vi "EventDrivenStateMachine.vi"() -> ()   [LabVIEW 2020]
panel:
  in  "Data2Tx":i32
  in  "Stop":bool
  in  "Tx":bool
  out "DataRx":i32
  in  "TxData":T1
  out "error out":errorcluster
  in  "error in":errorcluster
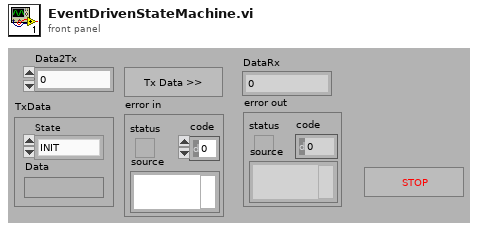
[diagram p1: front panel]
types:
  T1 = cluster{"Data":variant, "State":enum16{"INIT", "TX", "RX", "STOP"}}
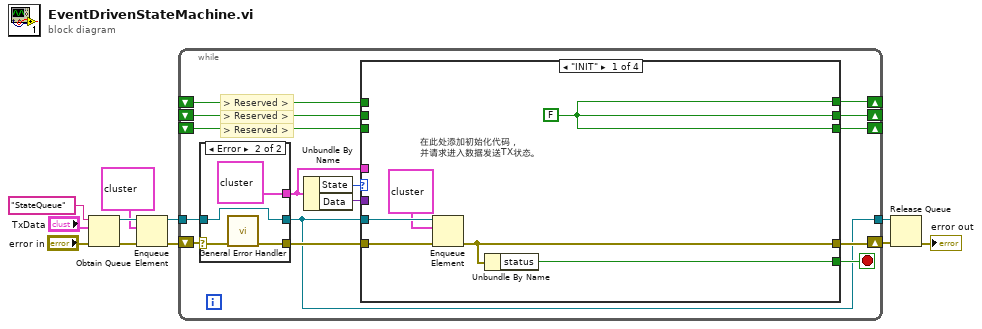
[diagram p0: block diagram]
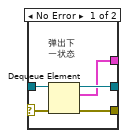
[diagram p2: hidden frame]
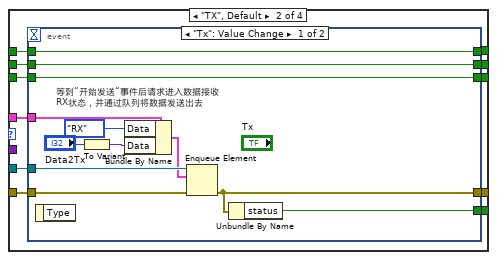
[diagram p3: hidden frame]
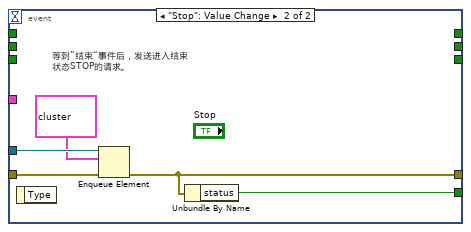
[diagram p4: hidden frame]
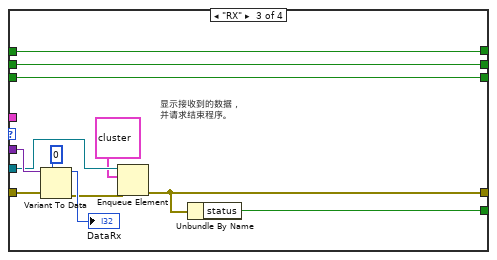
[diagram p5: hidden frame]
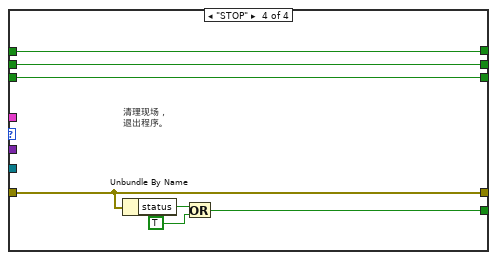
[diagram p6: hidden frame]
diagram:
  n1 = Obtain Queue(name (unnamed)="StateQueue", element data type="TxData", error in (no error)="error in") -> (queue out=w10:refnum<queue>, error out=w9:errorcluster)  [unwired: 2 in, 1 out]
  n2 = Enqueue Element(queue=w10, element=T1 {"Data"=variant, "State"=enum."INIT"} ("Queue Data"), error in (no error)=w9) -> (queue out=w3:refnum<queue>, error out=w2:errorcluster)  [unwired: 1 in, 1 out]
  n3 = while {
    shift-right: [w25] -> w8
    shift-left: w2 -> [w17]
    shift-right: [w21] -> _
    shift-left: _ -> [w19]
    shift-right: [w24] -> _
    shift-left: _ -> [w22]
    shift-right: [w23] -> _
    shift-left: _ -> [w20]
    tunnel: w3 -> [w18]
    tunnel: [w15] -> w7
    stop <- w26 stop-if-true
    # "> Reserved >"
    # "> Reserved >"
    # "> Reserved >"
    n4 = case shown="Error" w17 {
      selector: w17 -> [w30 w35]
      tunnel: w18 -> [w31 w34]
      tunnel: [w29 w34] -> w15
      tunnel: [w28 w33] -> w16
      tunnel: [w27 T1 {"Data"=variant, "State"=enum."RX"} ("Queue Data")] -> w12
      frame No Error {
        # "弹出下\n一状态"
        n5 = Dequeue Element(queue=w31, error in (no error)=w30) -> (queue out=w29:refnum<queue>, element=w27:T1, error out=w28:errorcluster)  [unwired: 1 in, 1 out]
      }
      frame Error {
        n6 = call <vilib>:"General Error Handler.vi"("error in (no error)"=w35) -> ("error out"=w33:errorcluster)  [unwired: 10 in, 4 out]
      }
    }
    n7 = Unbundle By Name(w12) -> ("State"=w14:enum16{"INIT", "TX", "RX", "STOP"}, "Data"=w13:variant)
    n8 = case shown="\"INIT\"" w14 {
      tunnel: [w40 w49 w78 w84] -> w26
      tunnel: w16 -> [w39 w52 w76 w85]
      tunnel: [w38 w50 w70 w85] -> w25
      tunnel: [w41 w43 w80 w87] -> w24
      tunnel: [w41 w42 w81 w86] -> w23
      tunnel: w22 -> [_ w46 w80 w87]
      tunnel: [w41 w44 w79 w88] -> w21
      tunnel: w20 -> [_ w45 w81 w86]
      tunnel: w19 -> [_ w47 w79 w88]
      tunnel: w15 -> [w37 w51 w72 _]
      tunnel: w13 -> [_ _ w77 _]
      tunnel: w12 -> [_ w48 _ _]
      frame "INIT" {
        w41 = FALSE
        # "在此处添加初始化代码，\n并请求进入数据发送TX状态。"
        n9 = Enqueue Element(queue=w37, element=T1 {"Data"=variant, "State"=enum."TX"} ("Queue Data"), error in (no error)=w39) -> (error out=w38:errorcluster)  [unwired: 1 in, 2 out]
        n10 = Unbundle By Name(w38) -> ("status"=w40:bool)
      }
      frame "TX", Default {
        n11 = event shown="[0] \"Tx\": Value Change" {
          selector: _ -> [_ _]
          dyn-events: _ -> [_ _]
          timeout: _ -> [_ _]
          tunnel: w52 -> [w64 w68]
          tunnel: w51 -> [w63 w69]
          tunnel: [w62 w65] -> w50
          tunnel: [w61 w66] -> w49
          tunnel: w48 -> [w60 _]
          tunnel: w47 -> [w57 _]
          tunnel: w46 -> [w56 _]
          tunnel: w45 -> [w55 _]
          tunnel: [w57 _] -> w44
          tunnel: [w56 _] -> w43
          tunnel: [w55 _] -> w42
          event "Tx": Value Change {
            # "等到“开始发送“事件后请求进入数据接收\nRX状态，并通过队列将数据发送出去"
            n12 = event-data() -> ()  [unwired: 1 in, 1 out]
            n13 = To Variant(anything="Data2Tx") -> (Variant=w58:variant)
            n14 = Bundle By Name(cluster=w60, "Data"=enum16{"INIT", "TX", "RX", "STOP"}."RX" ("State"), "Data"=w58) -> (w59:T1)
            n15 = Enqueue Element(queue=w63, element=w59, error in (no error)=w64) -> (error out=w62:errorcluster)  [unwired: 1 in, 2 out]
            n16 = Unbundle By Name(w62) -> ("status"=w61:bool)
          }
          event "Stop": Value Change {
            # "等到”结束“事件后，发送进入结束\n状态STOP的请求。"
            n17 = event-data() -> ()  [unwired: 1 in, 1 out]
            n18 = Enqueue Element(queue=w69, element=T1 {"Data"=variant, "State"=enum."STOP"} ("Queue Data"), error in (no error)=w68) -> (error out=w65:errorcluster)  [unwired: 1 in, 2 out]
            n19 = Unbundle By Name(w65) -> ("status"=w66:bool)
          }
        }
      }
      frame "RX" {
        # "显示接收到的数据，\n并请求结束程序。"
        n20 = Variant To Data(error in=w76, type=0, Variant=w77) -> (data=→"DataRx":i32, error out=w73:errorcluster)
        n21 = Enqueue Element(queue=w72, element=T1 {"Data"=variant, "State"=enum."TX"} ("Queue Data"), error in (no error)=w73) -> (error out=w70:errorcluster)  [unwired: 1 in, 2 out]
        n22 = Unbundle By Name(w70) -> ("status"=w78:bool)
      }
      frame "STOP" {
        # "清理现场，\n退出程序。"
        n23 = Unbundle By Name(w85) -> ("status"=w83:bool)
        n24 = Or(x=w83, y=TRUE ("x")) -> (x .or. y?=w84:bool)
      }
    }
  }
  n25 = Release Queue(queue=w7, error in (no error)=w8) -> (error out=→"error out":errorcluster)  [unwired: 1 in, 2 out]
